vi "xeva-checkTemperature.vi"(3 "error in (no error)":errorcluster, 5 "xeva-camref":T1) -> (0 "error out":errorcluster, 1 "xeva-temperature-reached":bool)   [LabVIEW 2015]
uses:
  <vilib>/Xenics Infrared Solutions/Xeneth LabVIEW API/VIs/Controls/Camara.ctl
  <vilib>/Xenics Infrared Solutions/Xeneth LabVIEW API/Xeneth.lvlib
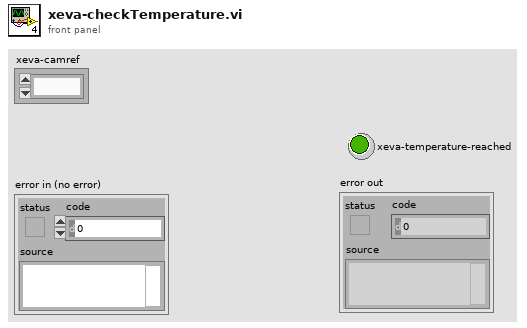
[diagram p1: front panel]
types:
  T1 = typedef "Xeneth.lvlib/Camara.ctl" = refnum<k1>
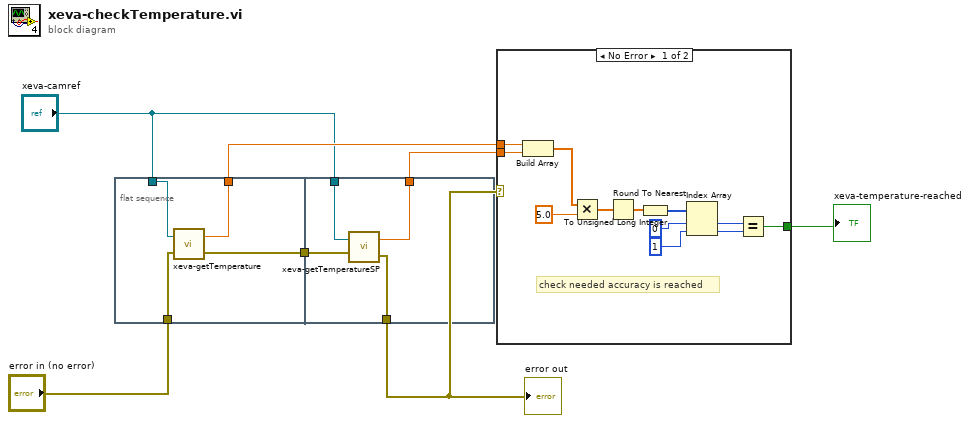
[diagram p0: block diagram]
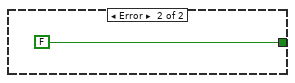
[diagram p2: hidden frame]
diagram:
  n1 = flat-sequence {
    tunnel: "xeva-camref" -> [w11]
    tunnel: "error in (no error)" -> [w10]
    tunnel: [w9] -> w5
    tunnel: [w8] -> w4
    tunnel: w5 -> [w14]
    tunnel: [w15] -> w1
    tunnel: "xeva-camref" -> [w13]
    tunnel: [w12] -> w2
    frame #0 {
      n2 = call "xeva-getTemperature.vi"("error in (no error)"=w10, "xeva-camref"=w11) -> ("error out"=w9:errorcluster, "xeva-temperature"=w8:dbl)
    }
    frame #1 {
      n3 = call "xeva-getTemperatureSP.vi"("error in (no error)"=w14, "xeva-camref"=w13) -> ("error out"=w15:errorcluster, "xeva-temperature-setpoint"=w12:dbl)
    }
  }
  n4 = case shown="No Error" w1 {
    tunnel: [w18 FALSE] -> w6
    tunnel: w4 -> [w17 _]
    tunnel: w2 -> [w16 _]
    frame No Error {
      # "check needed accuracy is reached"
      n5 = Build Array(w17, w16) -> (w25:dbl[])
      n6 = Multiply(x=w25, y=5.0) -> (x*y=w26:dbl[])
      n7 = Round To Nearest(number=w26) -> (nearest integer value=w24:dbl[])
      n8 = To Unsigned Long Integer(number=w24) -> (unsigned 32bit integer=w23:u32[])
      n9 = Index Array(array=w23, index #1=0 ("index"), index #2=1 ("index")) -> (element #1=w19:u32, element #2=w20:u32)
      n10 = Equal?(x=w19, y=w20) -> (x = y?=w18:bool)
    }
    frame Error {
    }
  }
  "xeva-temperature-reached" <- w6
  "error out" <- w1
